vi "WaitSingle.vi"(7 "wait option?":i32(ring) items=["MoveDone", "InPosition"], 8 "error in (no error)":errorcluster, 9 "timeout? (msec)":i32=-1, 10 "axis name":string, 11 "controller in":refnum<k24>) -> (0 "error out":errorcluster, 2 "completed":bool, 3 "controller out":refnum<k24>)   [LabVIEW 2020, in "Aerotech.lvlib"]
uses:
  Aerotech.lvlib
  C:/Users/HEP/Documents/GitHub/UCSB-Gantry-HEP/Drivers/Aerotech A3200/Bin/Aerotech.A3200.LabVIEW.dll
  UCSB-Gantry-HEP/Drivers/Aerotech A3200/Bin/Aerotech.A3200.LabVIEW.dll
  C:/Program Files (x86)/Aerotech/A3200/LabVIEW/2010/Bin/Aerotech.A3200.dll
  Program Files (x86)/Aerotech/A3200/LabVIEW/2010/Bin/Aerotech.A3200.dll
panel:
  in  "taskId":i32(ring) items=["TLibrary", "T01", "T02", "T03", "T04", "T05", "T06", "T07", "T08", "T09", "T10", "T11", "T12", "T13", "T14", "T15", "T16", "T17", "T18", "T19", "T20", "T21", "T22", "T23", "T24", "T25", "T26", "T27", "T28", "T29", "T30", "T31"]
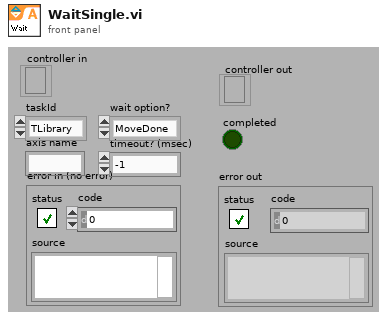
[diagram p1: front panel]
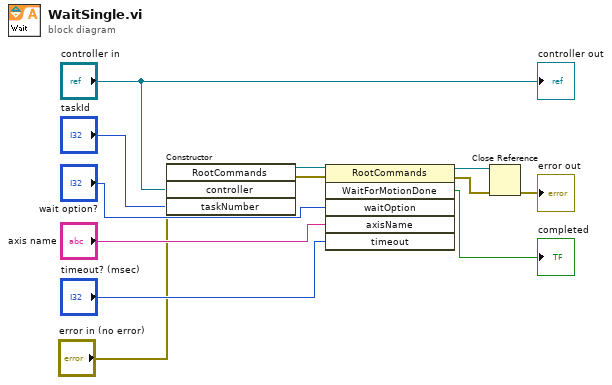
[diagram p0: block diagram]
diagram:
  n1 = constructor class="RootCommands"(error in="error in (no error)", "controller"="controller in", "taskNumber"="taskId") -> (reference out=w2:refnum<k24>, error out=w1:errorcluster)  [unwired: 2 in, 3 out]
  n2 = invoke class="RootCommands" method="WaitForMotionDone"(reference=w2, error in=w1, "waitOption"="wait option?", "axisName"="axis name", "timeout"="timeout? (msec)") -> (reference out=w7:refnum<k24>, error out=w8:errorcluster, "WaitForMotionDone"=→"completed":bool)  [unwired: 1 in, 3 out]
  n3 = Close Reference(reference=w7, error in (no error)=w8) -> (error out=→"error out":errorcluster)
  "controller out" <- "controller in"
